vi "Get Test Name.vi"(1 "board in":refnum<class "Board Design.lvclass">) -> (0 "test name":string)   [LabVIEW 2023, in "Board Design.lvclass"]
doc: "Build a test name for this class from the board class name and identification number."
uses:
  Board Design.lvclass
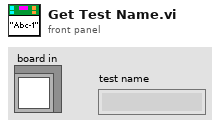
[diagram p1: front panel]
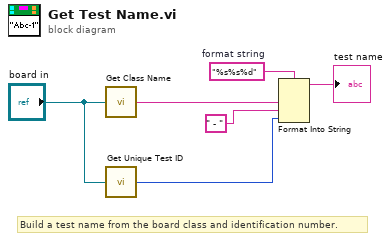
[diagram p0: block diagram]
diagram:
  w5 = "%s%s%d"  # format string
  # "Build a test name from the board class and identification number."
  n1 = call-dynamic "Get Class Name.vi"("board in"="board in") -> ("class name"=w4:string)
  n2 = call-dynamic "Get Unique Test ID.vi"("board in"="board in") -> ("id #"=w2:u32)
  n3 = Format Into String(format string=w5, w4, " - ", w2) -> (resulting string=→"test name":string)  [unwired: 2 in, 1 out]
